vi "Set Flow Rate.vi"(8 "error in (no error)":errorcluster, 9 "Flow Rate Units":T1, 10 "Flow Rate":dbl, 11 "Aalborg GFC17 in":refnum<class "Aalborg GFC17.lvclass">) -> (0 "error out":errorcluster, 3 "Aalborg GFC17 out":refnum<class "Aalborg GFC17.lvclass">)   [LabVIEW 2011, in "Aalborg GFC17.lvclass"]
uses:
  Aalborg GFC17.lvclass
  Mass Flow Controller/Flow Rate Units.ctl
  Aalborg GFC17.lvclass/Aalborg GFC17.ctl
  <vilib>/DAQmx/write.llb/DAQmx Write (Analog DBL 1Chan 1Samp).vi
  <vilib>/DAQmx/miscellaneous.llb/DAQmx Fill In Error Info.vi
  Mass Flow Controller/Mass Flow Controller.lvclass
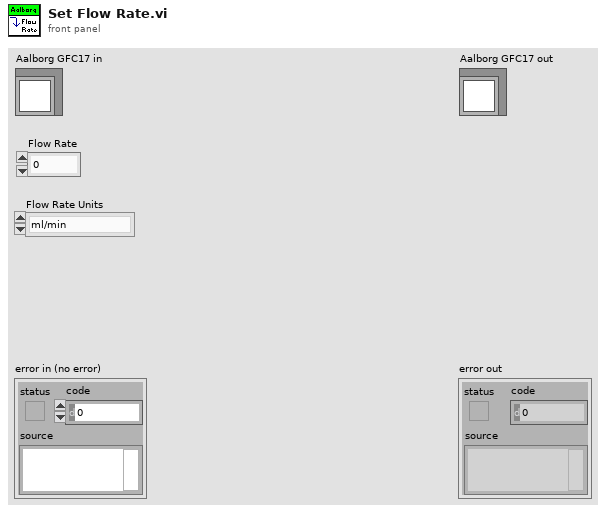
[diagram p1: front panel]
types:
  T1 = typedef "Mass Flow Controller.lvclass/Flow Rate Units.ctl" = enum16{"ml/min"}
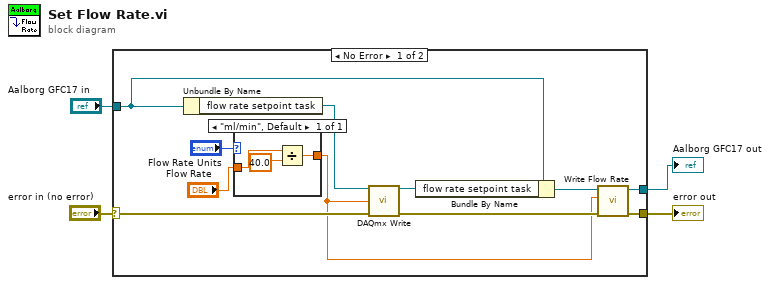
[diagram p0: block diagram]
diagram:
  n1 = case shown="No Error" "error in (no error)" {
    selector: "error in (no error)" -> [w10 w20]
    tunnel: [w7 w20] -> w3
    tunnel: [w6 w19] -> w1
    tunnel: "Aalborg GFC17 in" -> [w14 w19]
    frame No Error {
      n2 = Unbundle By Name(w14) -> ("flow rate setpoint task"=w15:refnum<k21>)
      n3 = case shown="\"ml/min\", Default" "Flow Rate Units" {
        tunnel: "Flow Rate" -> [w18]
        tunnel: [w16] -> w5
        frame "ml/min", Default {
          n4 = Divide(x=w18, y=40.0) -> (x/y=w16:dbl)
        }
      }
      n5 = call-poly <vilib>:"DAQmx Write.vi"("task/channels in"=w15, "data"=w5, "error in"=w10) -> ("task out"=w13:refnum<k21>, "error out"=w8:errorcluster)  [unwired: 10 in, 1 out]
      n6 = Bundle By Name(cluster=w14, "flow rate setpoint task"=w13) -> (w9:refnum<class "Aalborg GFC17.lvclass">)
      n7 = call-dynamic "Write Flow Rate.vi"("error in (no error)"=w8, "Flow Rate"=w5, "Mass Flow Controller in"=w9) -> ("error out"=w7:errorcluster, "Mass Flow Controller out"=w6:refnum<class "Aalborg GFC17.lvclass">)  [unwired: 7 in]
    }
    frame Error {
    }
  }
  "error out" <- w3
  "Aalborg GFC17 out" <- w1
